vi "afisaj_7seg.vi"() -> ()   [LabVIEW 2010]
panel:
  in  "stop":bool
  out "Slide":dbl(slide) scale=0.0..9.0
  out "L6":bool=TRUE
  out "L4":bool=TRUE
  out "L5":bool
  out "L7":bool=TRUE
  out "L3":bool=TRUE
  out "L2":bool=TRUE
  out "L1":bool=TRUE
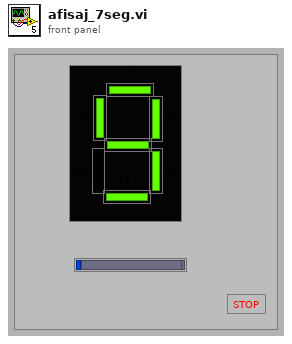
[diagram p1: front panel]
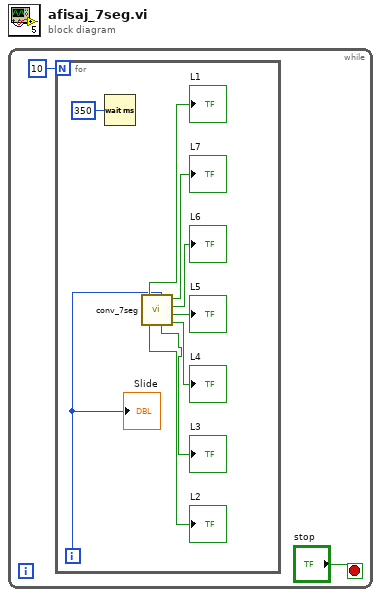
[diagram p0: block diagram]
diagram:
  n1 = while {
    stop <- "stop" stop-if-true
    n2 = for {
      N: 10 -> [_]
      i -> [w3]
      n3 = Wait (ms)(milliseconds to wait=u32 350) -> ()  [unwired: 1 out]
      n4 = call "conv_7seg.vi"("Numeric"=w3) -> ("Boolean 2"=→"L2":bool, "Boolean1"=→"L1":bool, "Boolean 3"=→"L3":bool, "Boolean 4"=→"L4":bool, "Boolean 5"=→"L5":bool, "Boolean 6"=→"L6":bool, "Boolean 7"=→"L7":bool)
      "Slide" <- w3
    }
  }
